vi "Create PV Data.vi"(8 "error in (no error)":errorcluster, 11 "NT Enum in":refnum<class "NT Enum.lvclass">) -> (0 "error out":errorcluster, 2 "PV Data out":refnum<class "PV Data.lvclass">, 3 "NT Enum out":refnum<class "NT Enum.lvclass">)   [LabVIEW 2020, in "PV Access.lvlib" / "PV Data.lvlib" / "NT Enum.lvclass"]
uses:
  NT Enum.lvclass
  PV Data/PV Data.lvclass
  NT Enum.lvclass/NT Enum.ctl
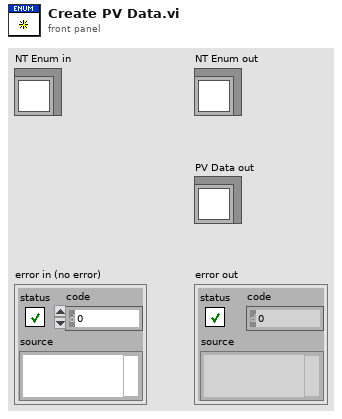
[diagram p1: front panel]
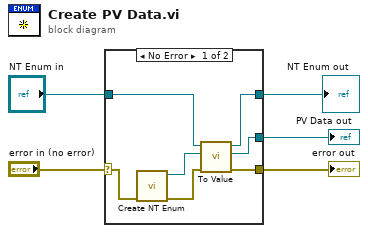
[diagram p0: block diagram]
diagram:
  n1 = case shown="No Error" "error in (no error)" {
    selector: "error in (no error)" -> [w12 w13]
    tunnel: "NT Enum in" -> [w11 w14]
    tunnel: [w10 w14] -> w3
    tunnel: [w6 w13] -> w2
    tunnel: [w8 _] -> w1
    frame No Error {
      n2 = call "Create NT Enum.vi"("error in"=w12) -> ("error out"=w7:errorcluster, "PV Data out"=w9:refnum<class "PV Data.lvclass">)  [unwired: 9 in]
      n3 = call-dynamic "To Value.vi"("error in (no error)"=w7, "PV Data in"=w9, "NT Enum in"=w11) -> ("error out"=w6:errorcluster, "PV Data out"=w8:refnum<class "PV Data.lvclass">, "NT Enum out"=w10:refnum<class "NT Enum.lvclass">)  [unwired: 6 in]
    }
    frame Error {
    }
  }
  "error out" <- w2
  "NT Enum out" <- w3
  "PV Data out" <- w1
